vi "Esercitazione 8 - Acquisizione ed elaborazione audio.vi"() -> ()   [LabVIEW 2018]
uses:
  <vilib>/sound2/lvsound2.llb/Sampling Mode.ctl
  <vilib>/sound2/lvsound2.llb/Sound Data Format.ctl
  <vilib>/sound2/lvsound2.llb/Sound Input Read (DBL).vi
  <vilib>/Waveform/WDTOps.llb/WDT Index Channel DBL.vi
panel:
  out "t0":timestamp[](array[timestamp])
  in  "stop":bool
  in  "Durata acquisizione":dbl
  out "Waveform Graph":waveform(dbl)(graph)
  in  "sound format":T1={"sample rate (S/s)"=22050.0, "number of channels"=2, "bits per sample"=16}
  in  "number of samples/ch":i32=100000
  in  "sample mode":T2=1 items=["Finite Samples", "Continuous Samples"]
  in  "device ID":u32
  # "la durata è data dal num. di campioni diviso\nla freq di campionamento, ovvero:\n10k/22050=0,453"
  # "per migliorare la funzionalità\nsi implementa una durata acquisizione esterna"
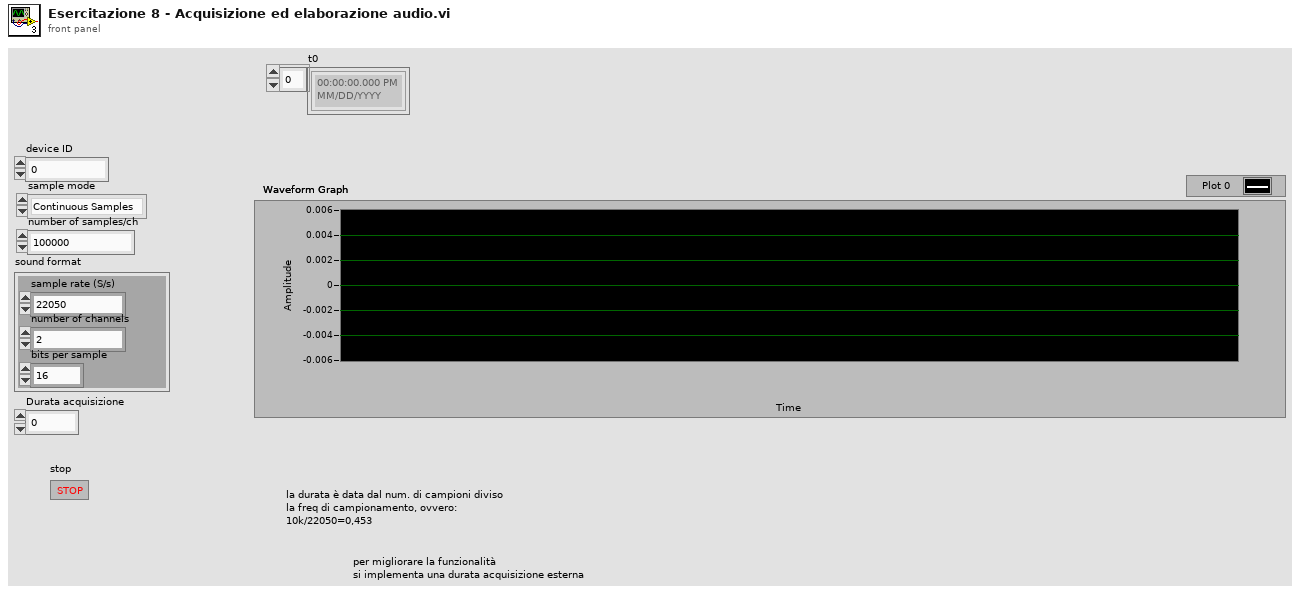
[diagram p1: front panel]
types:
  T1 = typedef "Sound Data Format.ctl" = cluster{"sample rate (S/s)":dbl, "number of channels":i32, "bits per sample":i32}
  T2 = typedef "Sampling Mode.ctl" = i32
  T3 = typedef "Sound Input Task ID.ctl" = u32
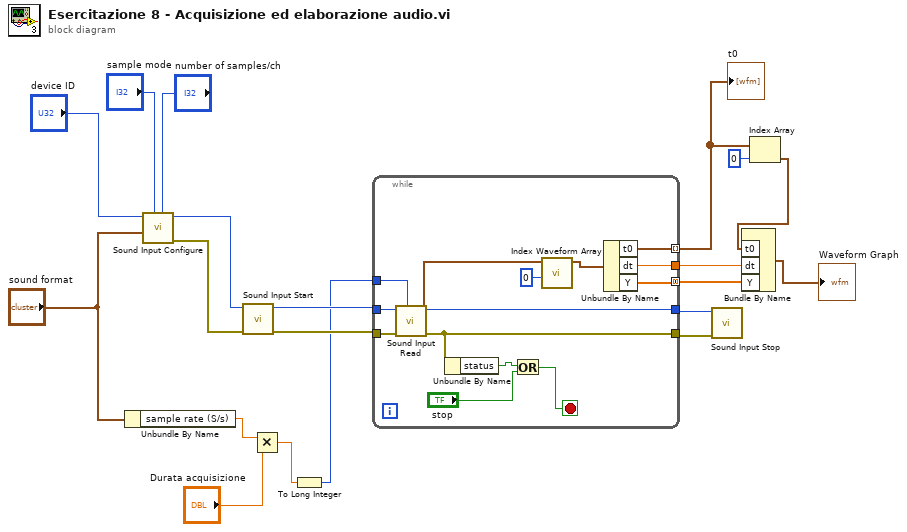
[diagram p0: block diagram]
diagram:
  n1 = Unbundle By Name("sound format") -> ("sample rate (S/s)"=w10:dbl)
  n2 = call <vilib>:"Sound Input Configure.vi"("number of samples/ch"="number of samples/ch", "sample mode"="sample mode", "sound format"="sound format", "device ID"="device ID") -> ("error out"=w19:errorcluster, "task ID"=w20:T3)  [unwired: 6 in]
  n3 = call <vilib>:"Sound Input Start.vi"("error in (no error)"=w19, "task ID"=w20) -> ("error out"=w14:errorcluster, "task ID out"=w15:T3)  [unwired: 8 in]
  n4 = Multiply(x=w10, y="Durata acquisizione") -> (x*y=w8:dbl)
  n5 = To Long Integer(number=w8) -> (32bit integer=w7:i32)
  n6 = while {
    tunnel: w7 -> [w31]
    tunnel: w15 -> [w34]
    tunnel: [w32] -> w13
    tunnel: w14 -> [w33]
    tunnel: [w30] -> w12
    tunnel: [w23] -> w5 mode=concatenating
    tunnel: [w22] -> w6
    tunnel: [w21] -> w3 mode=indexing
    stop <- w28 stop-if-true
    n7 = call-poly <vilib>:"Sound Input Read.vi"("number of samples/ch"=w31, "error in (no error)"=w33, "task ID"=w34) -> ("error out"=w30:errorcluster, "data"=w25:waveform(dbl)[], "task ID out"=w32:T3)  [unwired: 6 in]
    n8 = Unbundle By Name(w30) -> ("status"=w29:bool)
    n9 = Or(x=w29, y="stop") -> (x .or. y?=w28:bool)
    n10 = call-poly <vilib>:"Index Waveform Array.vi"("index"=0, "waveform array"=w25) -> ("waveform"=w24:waveform(dbl))  [unwired: 8 in, 1 out]
    n11 = Unbundle By Name(w24) -> ("t0"=w21:timestamp, "dt"=w22:dbl, "Y"=w23:dbl[])
  }
  "t0" <- w3
  n12 = call <vilib>:"Sound Input Stop.vi"("error in (no error)"=w12, "task ID"=w13) -> ()  [unwired: 8 in, 2 out]
  n13 = Index Array(array=w3, index=0) -> (element=w1:timestamp)
  n14 = Bundle By Name("t0"=w1, "dt"=w6, "Y"=w5) -> (→"Waveform Graph":waveform(dbl))  [unwired: 1 in]
